vi "capstone1 ver 4_mosfet.vi"() -> ()   [LabVIEW 2016]
uses:
  <instrlib>/Dynamixel Motor/Public/Motor Operation/Low Level/Baud Setting.ctl
  <vilib>/myRIO/Instrument Drivers/Onboard IO/DIO/typedefs/DIO Reference.ctl
  <vilib>/myRIO/Common/Instrument Driver Framework/Utilities/typedefs/myRIO Generic Hardware Reference.ctl
  <vilib>/myRIO/Common/Instrument Driver Framework/Utilities/typedefs/Hardware Version Enum.ctl
  <vilib>/myRIO/Common/Instrument Driver Framework/Utilities/typedefs/myRIO v1.0 Reference.ctl
  <vilib>/myRIO/Common/Instrument Driver Framework/Utilities/typedefs/Generic FPGA Reference.ctl
  <vilib>/myRIO/Common/Instrument Driver Framework/myRIO v1.0/DIO/typedefs/DIO Channels List.ctl
  <vilib>/myRIO/Common/Instrument Driver Framework/myRIO v1.0/DIO/typedefs/DIO Channels Enum.ctl
  <vilib>/userdefined/High Color/nirio_resource_hc.ctl
  <vilib>/myRIO/Common/Instrument Driver Framework/Utilities/vis/Is FPGA Ref Available.vi
  <vilib>/myRIO/Common/Instrument Driver Framework/myRIO v1.0/DIO/vis/myRIO v1.1 Open DIO.vi
  <vilib>/myRIO/Instrument Drivers/Onboard IO/DIO/vis/Write.vi
  <vilib>/myRIO/Common/Instrument Driver Framework/Utilities/vis/Validate Channels.vi
  <vilib>/myRIO/Common/Instrument Driver Framework/myRIO v1.0/DIO/vis/myRIO v1.0 Reserve DIO.vi
  <vilib>/myRIO/Instrument Drivers/Onboard IO/AO/vis/Write.vi
  <vilib>/myRIO/Common/Instrument Driver Framework/myRIO v1.0/Resource Manager/vis/myRIO v1.0 Reserve Channel List.vi
  <vilib>/myRIO/Common/Instrument Driver Framework/myRIO v1.0/DIO/vis/myRIO v1.0 Build MUX Configuration DIO.vi
  <vilib>/myRIO/Common/Instrument Driver Framework/myRIO v1.0/Resource Manager/vis/myRIO v1.0 Reserve Channel.vi
  <vilib>/myRIO/Common/Instrument Driver Framework/myRIO v1.0/Resource Manager/vis/myRIO v1.0 Unreserve Channel.vi
  <vilib>/myRIO/Common/Instrument Driver Framework/myRIO v1.0/Resource Manager/vis/myRIO v1.0 Create Configuration List.vi
  <vilib>/myRIO/Common/Instrument Driver Framework/myRIO v1.0/Resource Manager/vis/myRIO v1.0 Build Mutex Name.vi
  <vilib>/Utility/VariantDataType/GetNumericInfo.vi
  <vilib>/Utility/error.llb/Error Cluster From Error Code.vi
  <vilib>/myRIO/Common/Instrument Driver Framework/myRIO v1.0/myRIO v1.1 Open.vi
  <vilib>/myRIO/Common/Instrument Driver Framework/Utilities/vis/IO Manager.vi
  <vilib>/myRIO/Common/Instrument Driver Framework/Utilities/vis/Configuration Manager.vi
  <vilib>/myRIO/Common/Instrument Driver Framework/myRIO v1.0/Resource Manager/vis/myRIO v1.0 Configure IO.vi
  <vilib>/myRIO/Common/Instrument Driver Framework/myRIO v1.0/myRIO v1.0 Close.vi
  <vilib>/myRIO/Common/Instrument Driver Framework/myRIO v1.0/DIO/vis/myRIO v1.0 Write DIO.vi
  <vilib>/myRIO/Instrument Drivers/Onboard IO/AO/vis/Smart Open.vi
  <vilib>/myRIO/Common/Instrument Driver Framework/myRIO v1.0/AO/vis/myRIO v1.0 Write AO.vi
  <vilib>/myRIO/Express VI/Onboard Devices/LED/LED Express VI.xnode
  <vilib>/myRIO/Instrument Drivers/Onboard IO/DIO/vis/myRIO DIO Open.xnode
  <instrlib>/Dynamixel Motor/Dynamixel Motor.lvlib
  <vilib>/myRIO/Instrument Drivers/Onboard IO/DIO/DIO.lvlib
panel:
  out "motor temp":cluster{"0":sgl, "1":sgl, "2":sgl, "3":sgl}
  out "value":T1
  out "TCP Read data":string
  in  "정지":bool
  out "error out":errorcluster
  out "RT TCP Loop time":u32
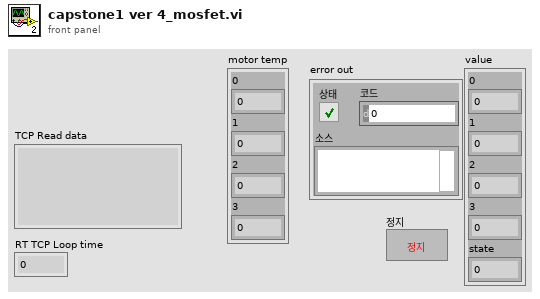
[diagram p1: front panel]
types:
  T1 = cluster{"0":sgl, "1":sgl, "2":sgl, "3":sgl, "state":sgl}
  T2 = typedef "Dynamixel Motor.lvlib/Baud Setting.ctl" = u8
  T3 = enum16{"big-endian, network order", "native, host order", "little-endian"}
  T4 = cluster{"0":sgl, "1":sgl, "2":sgl, "3":sgl, "state":i32}
  T5 = typedef "DIO.lvlib/DIO Reference.ctl" = cluster{"myRIO Reference":T6, "DIO Channels List":T10}
  T6 = typedef "myRIO Generic Hardware Reference.ctl" = cluster{"myRIO Model":T7, "myRIO Hardware Reference":T8}
  T7 = typedef "Hardware Version Enum.ctl" = enum16{"Unknown", "myRIO-1900", "myRIO-1950", "roboRIO", "NI ELVIS RIO CM"}
  T8 = typedef "myRIO v1.0 Reference.ctl" = cluster{"Generic FPGA Reference":T9, "Allow multiple opens":bool}
  T9 = typedef "Generic FPGA Reference.ctl" = refnum<k20>
  T10 = typedef "DIO Channels List.ctl" = T11[]
  T11 = typedef "DIO Channels Enum.ctl" = enum16{"Not Connected", "C/DIO0", "C/DIO1", "C/DIO2", "C/DIO3", "C/DIO4", "C/DIO5", "C/DIO6", "C/DIO7", "A/DIO0", "A/DIO1", "A/DIO2", "A/DIO3", "A/DIO4", "A/DIO5", "A/DIO6", "A/DIO7", "A/DIO8", "A/DIO9", "A/DIO10", "A/DIO11", "A/DIO12", "A/DIO13", "A/DIO14", "A/DIO15", "B/DIO0", "B/DIO1", "B/DIO2", "B/DIO3", "B/DIO4", "B/DIO5", "B/DIO6", "B/DIO7", "B/DIO8", "B/DIO9", "B/DIO10", "B/DIO11", "B/DIO12", "B/DIO13", "B/DIO14", "B/DIO15", "LED0", "LED1", "LED2", "LED3", "Button0", "DIO/DIO0", "DIO/DIO1", "DIO/DIO2", "DIO/DIO3", "DIO/DIO4", "DIO/DIO5", "DIO/DIO6", "DIO/DIO7", "DIO/DIO8", "DIO/DIO9", "SPI/CS0", "SPI/CS1", "SPI/CS2", "SPI/CS3", "LED RADIO (Green)", "LED RADIO (Red)", "LED COMM (Green)", "LED COMM (Red)", "LED MODE (Green)", "LED MODE (Red)"}
  T12 = typedef "nirio_resource_hc.ctl" = tag
  T13 = cluster{"Temperature (C)":u8, "Temperature (C)":u8, "Temperature (C)":u8, "Temperature (C)":u8}
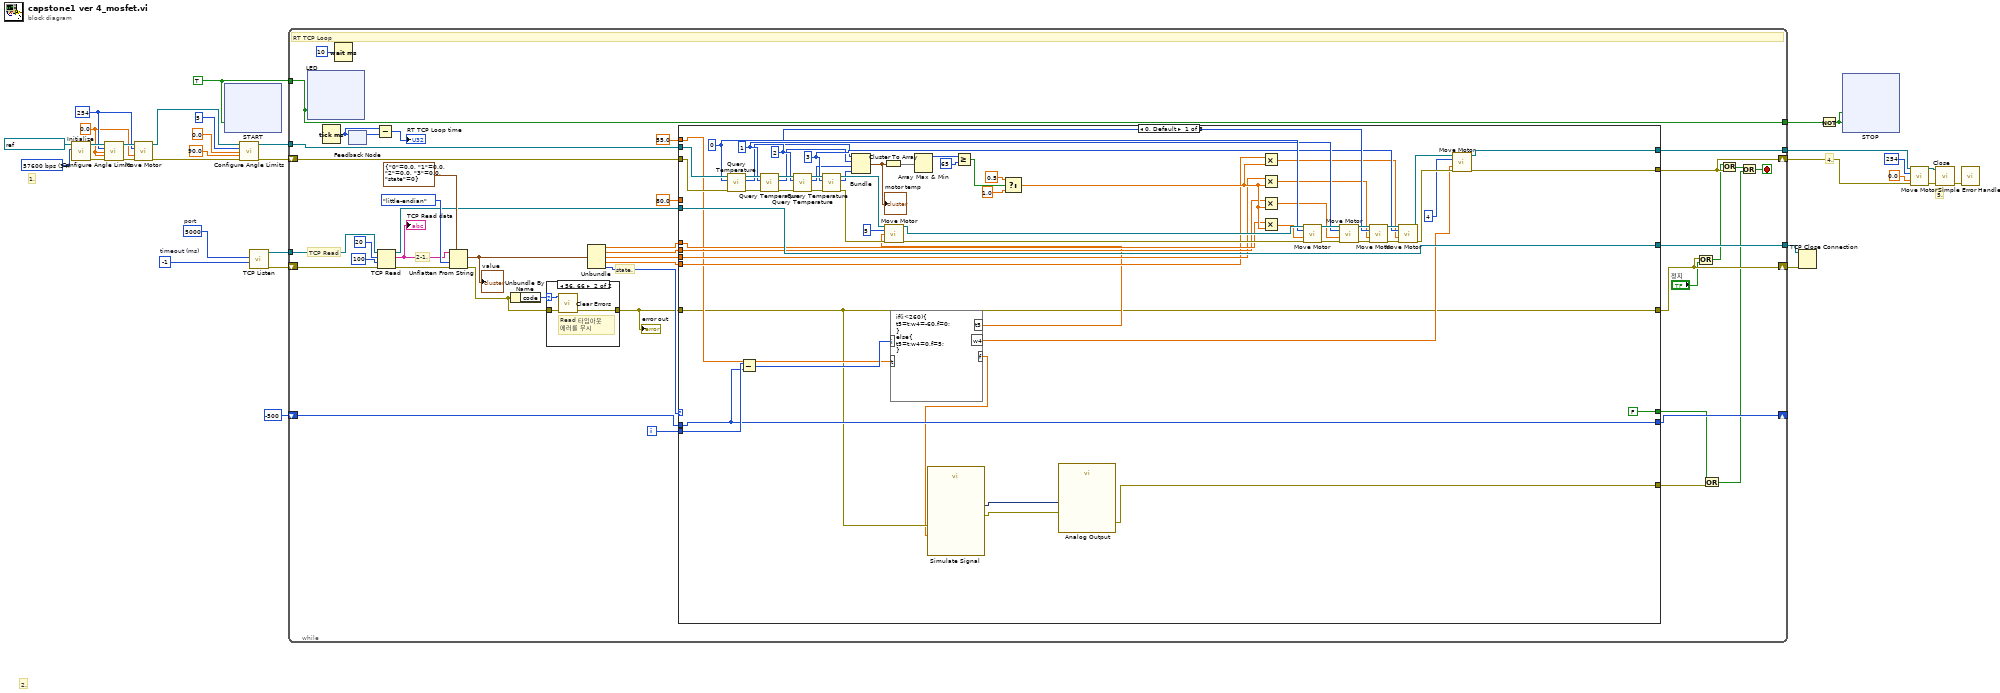
[diagram p0: block diagram]
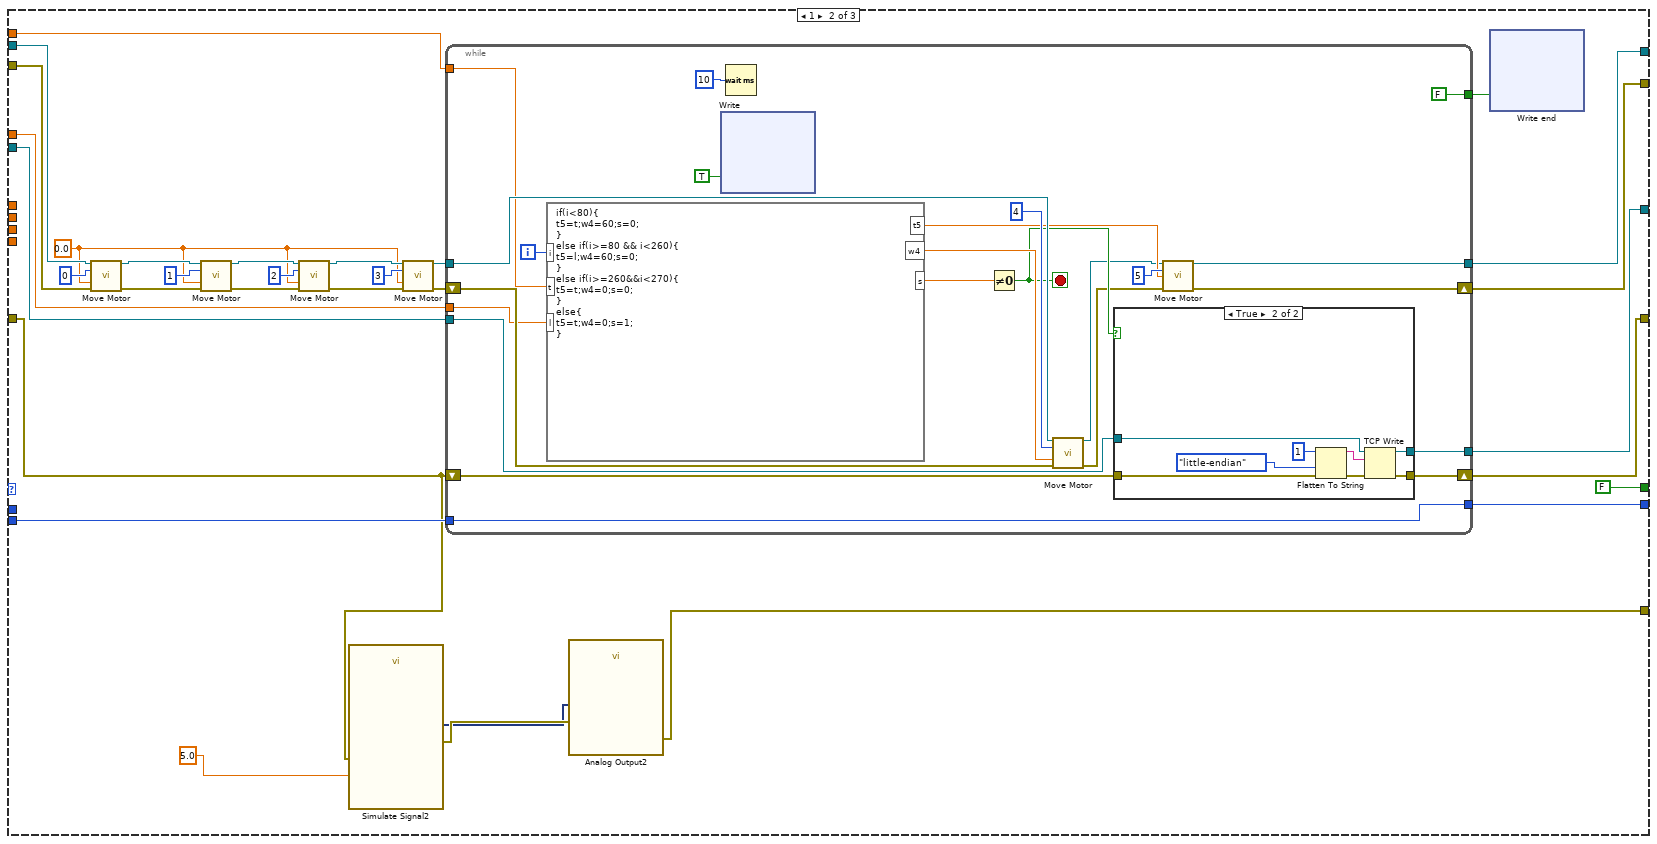
[diagram p2: hidden frame]
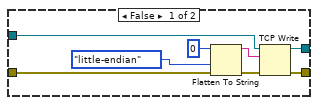
[diagram p3: hidden frame]
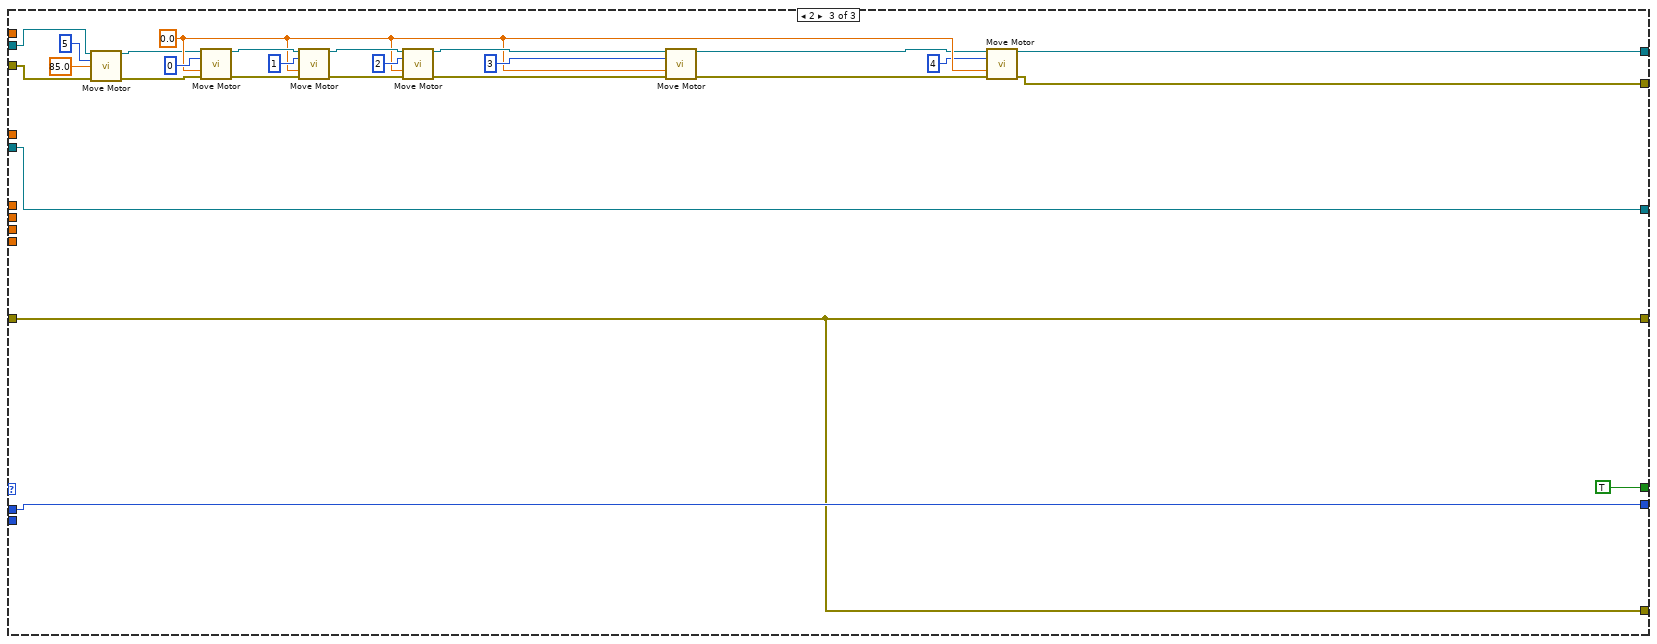
[diagram p4: hidden frame]
diagram:
  w26 = T2 34 items=["1,000,000 bps"=1, "500,000 bps"=3, "400,000 bps"=4, "250,000 bps"=7, "200,000 bps"=9, "115200 bps"=16, "57600 bps"=34, "19200 bps"=103, "9600 bps"=207] ("Baud rate (57600 bps)")
  w9 = TRUE
  w11 = u8 254 ("Motor ID (0)")
  w10 = 0.0 ("Clockwise Angle Limit (0 deg)")
  w31 = u16 5000  # port
  w32 = -1  # timeout (ms)
  # "5."
  # "4."
  # "2."
  # "1."
  n1 = call <instrlib>:"Initialize.vi"("Baud rate (57600 bps)"=w26, "VISA resource name"=refnum<visa-resource-name> "ASRL3::INSTR") -> ("error out"=w20:errorcluster, "VISA resource name out"=w19:refnum<visa-resource-name>)  [unwired: 8 in]
  n2 = call <instrlib>:"Configure Angle Limits.vi"("VISA resource name"=w19, "Motor ID (0)"=w11, "Clockwise Angle Limit (0 deg)"=w10, "Counter-Clockwise Angle Limit (300 deg)"=w10, "error in (no error)"=w20) -> ("VISA resource name out"=w13:refnum<visa-resource-name>, "error out"=w12:errorcluster)  [unwired: 9 in]
  n3 = call <instrlib>:"Move Motor.vi"("VISA resource name"=w13, "Motor ID (0)"=w11, "Goal Speed (RPM)"=w10, "error in (no error)"=w12) -> ("VISA resource name out"=w7:refnum<visa-resource-name>, "error out"=w8:errorcluster)  [unwired: 10 in]
  n4 = xnode "START"("LED0"=w9) -> ()  [unwired: 1 in, 1 out]
  n5 = call <instrlib>:"Configure Angle Limits.vi"("VISA resource name"=w7, "Motor ID (0)"=5, "Clockwise Angle Limit (0 deg)"=0.0, "Counter-Clockwise Angle Limit (300 deg)"=90.0 ("Clockwise Angle Limit (0 deg)"), "error in (no error)"=w8) -> ("VISA resource name out"=w16:refnum<visa-resource-name>, "error out"=w2:errorcluster)  [unwired: 9 in]
  n6 = call <vilib>:"TCP Listen.vi"("timeout ms (wait forever: -1)"=w32, "port"=w31) -> ("error out"=w27:errorcluster, "connection ID"=w28:refnum<k5>)  [unwired: 5 in, 3 out]
  n7 = while {
    tunnel: w28 -> [w60]
    tunnel: [w51] -> w30
    shift-right: [w47] -> w29
    shift-left: w27 -> [w61]
    shift-right: [w46] -> w6
    shift-left: w2 -> [w40]
    tunnel: w9 -> [w59]
    tunnel: [w59] -> w22
    tunnel: w16 -> [w49]
    tunnel: [w48] -> w5
    shift-right: [w37] -> _
    shift-left: -500 -> [w36]
    i -> [w38]
    stop <- w42 stop-if-true
    # "state."
    # "2-1."
    # "TCP Read"
    # "RT TCP Loop"
    n8 = xnode "LED"("LED1"=w59) -> ()  [unwired: 1 in, 1 out]
    n9 = Tick Count (ms)() -> (millisecond timer value=w70:u32)
    n10 = Wait (ms)(milliseconds to wait=u32 10 ("대기 시간 (ms)")) -> ()  [unwired: 1 out]
    n11 = feedback #1() -> (w71:u32)  [unwired: 1 in]
    n12 = feedback-in #1(w70) -> ()
    n13 = Subtract(x=w70, y=w71) -> (x-y=→"RT TCP Loop time":u32)
    n14 = TCP Read(connection ID=w60, bytes to read=20 ("읽을 바이트"), error in (no error)=w61, 9:100 ("타임아웃 ms (25000)")) -> (connection ID out=w52:refnum<k5>, data out=w64:string, error out=w63:errorcluster)  [unwired: 1 in]
    "TCP Read data" <- w64
    n15 = Unflatten From String(type=T4 {"0"=0.0, "1"=0.0, "2"=0.0, "3"=0.0, "state"=0}, binary string=w64, byte order (0:big-endian, network order)=T3."little-endian", error in (no error)=w63) -> (value=w58:T4, error out=w62:errorcluster)  [unwired: 1 in, 1 out]
    "value" <- w58
    n16 = Unbundle By Name(w62) -> ("code"=w72:i32)
    n17 = case shown="56, 66" w72 {
      selector: w72 -> [_ w338]
      tunnel: [w336 w337] -> w50
      tunnel: w62 -> [w336 w339]
      frame 0, Default {
      }
      frame 56, 66 {
        # "Read 타임아웃\n에러를 무시"
        n18 = call <vilib>:"Clear Errors.vi"("error in (no error)"=w339, "specific error code to clear (0: all)"=w338) -> ("error out"=w337:errorcluster)  [unwired: 4 in, 1 out]
      }
    }
    "error out" <- w50
    n19 = Unbundle(w58) -> ("0"=w57:sgl, "1"=w55:sgl, "2"=w56:sgl, "3"=w54:sgl, "state"=w53:i32)
    n20 = case shown="0, Default" w53 {
      tunnel: w57 -> [w102 _ _]
      tunnel: w55 -> [w100 _ _]
      tunnel: w56 -> [w98 _ _]
      tunnel: w54 -> [w96 _ _]
      tunnel: w49 -> [w115 w155 w280]
      tunnel: [w126 w150 w287] -> w48
      tunnel: [w124 w151 w286] -> w46
      tunnel: w40 -> [w86 w145 w283]
      tunnel: w52 -> [w122 w149 w282]
      tunnel: [w122 w147 w282] -> w51
      tunnel: w50 -> [w78 w137 w275]
      tunnel: [w78 w148 w275] -> w47
      tunnel: 55.0 -> [w81 w144 _]
      tunnel: 80.0 -> [_ w143 _]
      tunnel: [FALSE FALSE TRUE] -> w34
      tunnel: w38 -> [w84 w141 _]
      tunnel: [w83 w140 w276] -> w37
      tunnel: w36 -> [w83 _ w276]
      tunnel: [w76 w136 w275] -> w35
      frame 0, Default {
        w110 = 3
        w111 = 2
        w112 = 1
        w113 = 0
        n21 = call <instrlib>:"Query Temperature.vi"("error in"=w86, "Motor ID (0)"=w113, "VISA resource name"=w115) -> ("error out"=w109:errorcluster, "Temperature (C)"=w94:u8, "VISA resource name out"=w118:refnum<visa-resource-name>)  [unwired: 6 in]
        n22 = Subtract(x=w84, y=w83) -> (x-y=w82:i32)
        n23 = call <instrlib>:"Query Temperature.vi"("error in"=w109, "Motor ID (0)"=w112, "VISA resource name"=w118) -> ("error out"=w108:errorcluster, "Temperature (C)"=w93:u8, "VISA resource name out"=w117:refnum<visa-resource-name>)  [unwired: 6 in]
        n24 = call <instrlib>:"Query Temperature.vi"("error in"=w108, "Motor ID (0)"=w111, "VISA resource name"=w117) -> ("error out"=w107:errorcluster, "Temperature (C)"=w92:u8, "VISA resource name out"=w116:refnum<visa-resource-name>)  [unwired: 6 in]
        n25 = call <instrlib>:"Query Temperature.vi"("error in"=w107, "Motor ID (0)"=w110, "VISA resource name"=w116) -> ("error out"=w85:errorcluster, "Temperature (C)"=w91:u8, "VISA resource name out"=w114:refnum<visa-resource-name>)  [unwired: 6 in]
        n26 = Bundle("Temperature (C)"=w94, "Temperature (C)"=w93, "Temperature (C)"=w92, "Temperature (C)"=w91) -> (w88:T13)  [unwired: 1 in]
        "motor temp" <- w88
        n27 = Cluster To Array(cluster=w88) -> (array=w90:u8[])
        n28 = formula code="if(i<260){\nt5=t;w4=-60,f=0;\n}\nelse{\nt5=t;w4=0,f=5;\n}"("i"=w82, "t"=w81) -> ("t5"=w80:dbl, "w4"=w79:dbl, "f"=w74:dbl)
        n29 = call <instrlib>:"Move Motor.vi"("VISA resource name"=w114, "Motor ID (0)"=5, "Goal Position (180 deg)"=w80, "error in (no error)"=w85) -> ("VISA resource name out"=w120:refnum<visa-resource-name>, "error out"=w121:errorcluster)  [unwired: 10 in]
        n30 = Array Max & Min(array=w90) -> (max value=w89:u8)  [unwired: 3 out]
        n31 = call "Simulate Signal"("Offset"=w74, "error in (no error)"=w78) -> ("DC"=w75:dynamicdata, "error out"=w77:errorcluster)  [unwired: 12 in]
        n32 = Greater Or Equal?(x=w89, y=65) -> (x >= y?=w87:bool)
        n33 = Select(t=0.5, s=w87, f=1.0) -> (s? t:f=w103:dbl)
        n34 = call "Analog Output"("AudioOut/Right"=w75, "error in (no error)"=w77) -> ("error out"=w76:errorcluster)  [unwired: 25 in]
        n35 = Multiply(x=w96, y=w103) -> (x*y=w95:dbl)
        n36 = Multiply(x=w98, y=w103) -> (x*y=w97:dbl)
        n37 = Multiply(x=w100, y=w103) -> (x*y=w99:dbl)
        n38 = Multiply(x=w102, y=w103) -> (x*y=w101:dbl)
        n39 = call <instrlib>:"Move Motor.vi"("VISA resource name"=w120, "Motor ID (0)"=w113, "Goal Speed (RPM)"=w101, "error in (no error)"=w121) -> ("VISA resource name out"=w129:refnum<visa-resource-name>, "error out"=w130:errorcluster)  [unwired: 10 in]
        n40 = call <instrlib>:"Move Motor.vi"("VISA resource name"=w129, "Motor ID (0)"=w112, "Goal Speed (RPM)"=w99, "error in (no error)"=w130) -> ("VISA resource name out"=w131:refnum<visa-resource-name>, "error out"=w133:errorcluster)  [unwired: 10 in]
        n41 = call <instrlib>:"Move Motor.vi"("VISA resource name"=w131, "Motor ID (0)"=w111, "Goal Speed (RPM)"=w97, "error in (no error)"=w133) -> ("VISA resource name out"=w132:refnum<visa-resource-name>, "error out"=w134:errorcluster)  [unwired: 10 in]
        n42 = call <instrlib>:"Move Motor.vi"("VISA resource name"=w132, "Motor ID (0)"=w110, "Goal Speed (RPM)"=w95, "error in (no error)"=w134) -> ("VISA resource name out"=w127:refnum<visa-resource-name>, "error out"=w125:errorcluster)  [unwired: 10 in]
        n43 = call <instrlib>:"Move Motor.vi"("VISA resource name"=w127, "Motor ID (0)"=4, "Goal Speed (RPM)"=w79, "error in (no error)"=w125) -> ("VISA resource name out"=w126:refnum<visa-resource-name>, "error out"=w124:errorcluster)  [unwired: 10 in]
      }
      frame 1 {
        w154 = 0.0
        n44 = call <instrlib>:"Move Motor.vi"("VISA resource name"=w155, "Motor ID (0)"=0, "Goal Speed (RPM)"=w154, "error in (no error)"=w145) -> ("VISA resource name out"=w156:refnum<visa-resource-name>, "error out"=w157:errorcluster)  [unwired: 10 in]
        n45 = call <instrlib>:"Move Motor.vi"("VISA resource name"=w156, "Motor ID (0)"=1, "Goal Speed (RPM)"=w154, "error in (no error)"=w157) -> ("VISA resource name out"=w158:refnum<visa-resource-name>, "error out"=w160:errorcluster)  [unwired: 10 in]
        n46 = call <instrlib>:"Move Motor.vi"("VISA resource name"=w158, "Motor ID (0)"=2, "Goal Speed (RPM)"=w154, "error in (no error)"=w160) -> ("VISA resource name out"=w159:refnum<visa-resource-name>, "error out"=w161:errorcluster)  [unwired: 10 in]
        n47 = call "Simulate Signal2"("Offset"=5.0, "error in (no error)"=w137) -> ("DC"=w135:dynamicdata, "error out"=w138:errorcluster)  [unwired: 12 in]
        n48 = call <instrlib>:"Move Motor.vi"("VISA resource name"=w159, "Motor ID (0)"=3, "Goal Speed (RPM)"=w154, "error in (no error)"=w161) -> ("VISA resource name out"=w152:refnum<visa-resource-name>, "error out"=w153:errorcluster)  [unwired: 10 in]
        n49 = while {
          shift-right: [w208] -> w151
          shift-left: w153 -> [w221]
          shift-right: [w213] -> w148
          shift-left: w137 -> [w214]
          tunnel: w149 -> [w215]
          tunnel: [w212] -> w147
          tunnel: [FALSE] -> w146
          tunnel: w152 -> [w222]
          tunnel: [w209] -> w150
          tunnel: w144 -> [w205]
          tunnel: w143 -> [w204]
          tunnel: [w201] -> w140
          tunnel: w141 -> [w201]
          i -> [w219]
          stop <- w216 stop-if-true
          n50 = formula code="if(i<80){\nt5=t;w4=60;s=0;\n}\nelse if(i>=80 && i<260){\nt5=l;w4=60;s=0;\n}\nelse if(i>=260&&i<270){\nt5=t;w4=0;s=0;\n}\nelse{\nt5=t;w4=0;s=1;\n}"("i"=w219, "t"=w205, "l"=w204) -> ("t5"=w206:dbl, "w4"=w218:dbl, "s"=w217:dbl)
          n51 = xnode "Write"("LED2"=TRUE) -> ()  [unwired: 1 in, 1 out]
          n52 = Wait (ms)(milliseconds to wait=u32 10 ("대기 시간 (ms)")) -> ()  [unwired: 1 out]
          n53 = Not Equal To 0?(x=w217) -> (x != 0?=w216:bool)
          n54 = call <instrlib>:"Move Motor.vi"("VISA resource name"=w222, "Motor ID (0)"=4, "Goal Speed (RPM)"=w218, "error in (no error)"=w221) -> ("VISA resource name out"=w203:refnum<visa-resource-name>, "error out"=w202:errorcluster)  [unwired: 10 in]
          n55 = case shown="True" w216 {
            tunnel: w215 -> [w262 w274]
            tunnel: [w260 w270] -> w212
            tunnel: w214 -> [w261 w269]
            tunnel: [w259 w267] -> w213
            frame False {
              n56 = Flatten To String(anything=0, byte order (0:big-endian, network order)=T3."little-endian", error in (no error)=w261) -> (data string=w264:string, error out=w263:errorcluster)  [unwired: 1 in, 1 out]
              n57 = TCP Write(connection ID=w262, data in=w264, error in (no error)=w263) -> (connection ID out=w260:refnum<k5>, error out=w259:errorcluster)  [unwired: 1 in, 1 out]
            }
            frame True {
              n58 = Flatten To String(anything=1, byte order (0:big-endian, network order)=T3."little-endian", error in (no error)=w269) -> (data string=w271:string, error out=w268:errorcluster)  [unwired: 1 in, 1 out]
              n59 = TCP Write(connection ID=w274, data in=w271, error in (no error)=w268) -> (connection ID out=w270:refnum<k5>, error out=w267:errorcluster)  [unwired: 1 in, 1 out]
            }
          }
          n60 = call <instrlib>:"Move Motor.vi"("VISA resource name"=w203, "Motor ID (0)"=5, "Goal Position (180 deg)"=w206, "error in (no error)"=w202) -> ("VISA resource name out"=w209:refnum<visa-resource-name>, "error out"=w208:errorcluster)  [unwired: 10 in]
        }
        n61 = call "Analog Output2"("AudioOut/Right"=w135, "error in (no error)"=w138) -> ("error out"=w136:errorcluster)  [unwired: 25 in]
        n62 = xnode "Write end"("LED2"=w146) -> ()  [unwired: 1 in, 1 out]
      }
      frame 2 {
        w290 = 0.0
        n63 = call <instrlib>:"Move Motor.vi"("VISA resource name"=w280, "Motor ID (0)"=5, "Goal Position (180 deg)"=85.0, "error in (no error)"=w283) -> ("VISA resource name out"=w279:refnum<visa-resource-name>, "error out"=w281:errorcluster)  [unwired: 10 in]
        n64 = call <instrlib>:"Move Motor.vi"("VISA resource name"=w279, "Motor ID (0)"=0, "Goal Speed (RPM)"=w290, "error in (no error)"=w281) -> ("VISA resource name out"=w300:refnum<visa-resource-name>, "error out"=w299:errorcluster)  [unwired: 10 in]
        n65 = call <instrlib>:"Move Motor.vi"("VISA resource name"=w300, "Motor ID (0)"=1, "Goal Speed (RPM)"=w290, "error in (no error)"=w299) -> ("VISA resource name out"=w298:refnum<visa-resource-name>, "error out"=w296:errorcluster)  [unwired: 10 in]
        n66 = call <instrlib>:"Move Motor.vi"("VISA resource name"=w298, "Motor ID (0)"=2, "Goal Speed (RPM)"=w290, "error in (no error)"=w296) -> ("VISA resource name out"=w297:refnum<visa-resource-name>, "error out"=w295:errorcluster)  [unwired: 10 in]
        n67 = call <instrlib>:"Move Motor.vi"("VISA resource name"=w297, "Motor ID (0)"=3, "Goal Speed (RPM)"=w290, "error in (no error)"=w295) -> ("VISA resource name out"=w288:refnum<visa-resource-name>, "error out"=w285:errorcluster)  [unwired: 10 in]
        n68 = call <instrlib>:"Move Motor.vi"("VISA resource name"=w288, "Motor ID (0)"=4, "Goal Speed (RPM)"=w290, "error in (no error)"=w285) -> ("VISA resource name out"=w287:refnum<visa-resource-name>, "error out"=w286:errorcluster)  [unwired: 10 in]
      }
    }
    n69 = Or(x=w47, y="정지") -> (x .or. y?=w39:bool)
    n70 = Or(x=w34, y=w35) -> (x .or. y?=w33:bool)
    n71 = Or(x=w39, y=w46) -> (x .or. y?=w43:bool)
    n72 = Or(x=w43, y=w33) -> (x .or. y?=w42:bool)
  }
  n73 = TCP Close Connection(connection ID=w30, error in (no error)=w29) -> ()  [unwired: 3 out]
  n74 = Not(x=w22) -> (.not. x?=w21:bool)
  n75 = xnode "STOP"("LED0"=w21, "LED1"=w21) -> ()  [unwired: 1 in, 1 out]
  n76 = call <instrlib>:"Move Motor.vi"("VISA resource name"=w5, "Motor ID (0)"=u8 254, "Goal Speed (RPM)"=0.0, "error in (no error)"=w6) -> ("VISA resource name out"=w4:refnum<visa-resource-name>, "error out"=w3:errorcluster)  [unwired: 10 in]
  n77 = call <instrlib>:"Close.vi"("error in (no error)"=w3, "VISA resource name"=w4) -> ("error out"=w15:errorcluster)  [unwired: 9 in]
  n78 = call <vilib>:"Simple Error Handler.vi"("error in (no error)"=w15) -> ()  [unwired: 4 in, 5 out]
